vi "OEE_SCREEN_1_edit_running_summary.vi"(8 "error_in":errorcluster, 11 "running_summary":string) -> (0 "error_out":errorcluster, 3 "running_summary_updated":string)   [LabVIEW 2019]
uses:
  FGV/SQL_connection/FGV_OEE_SQL_connection.ctl
  FGV/SQL_raw_data/FGV_OEE_SQL_raw_data.ctl
  _misc/AULocalize/SubVIs/RegisterVI.vi
  _misc/AULocalize/SubVIs/Get Localized Phrase Compact Interface 0D.vi
panel:
  in  "summary_edit_cancel":bool caption="cancel"
  in  "summary_edit_update":bool caption="update"
  in  "running_summary_editor":string
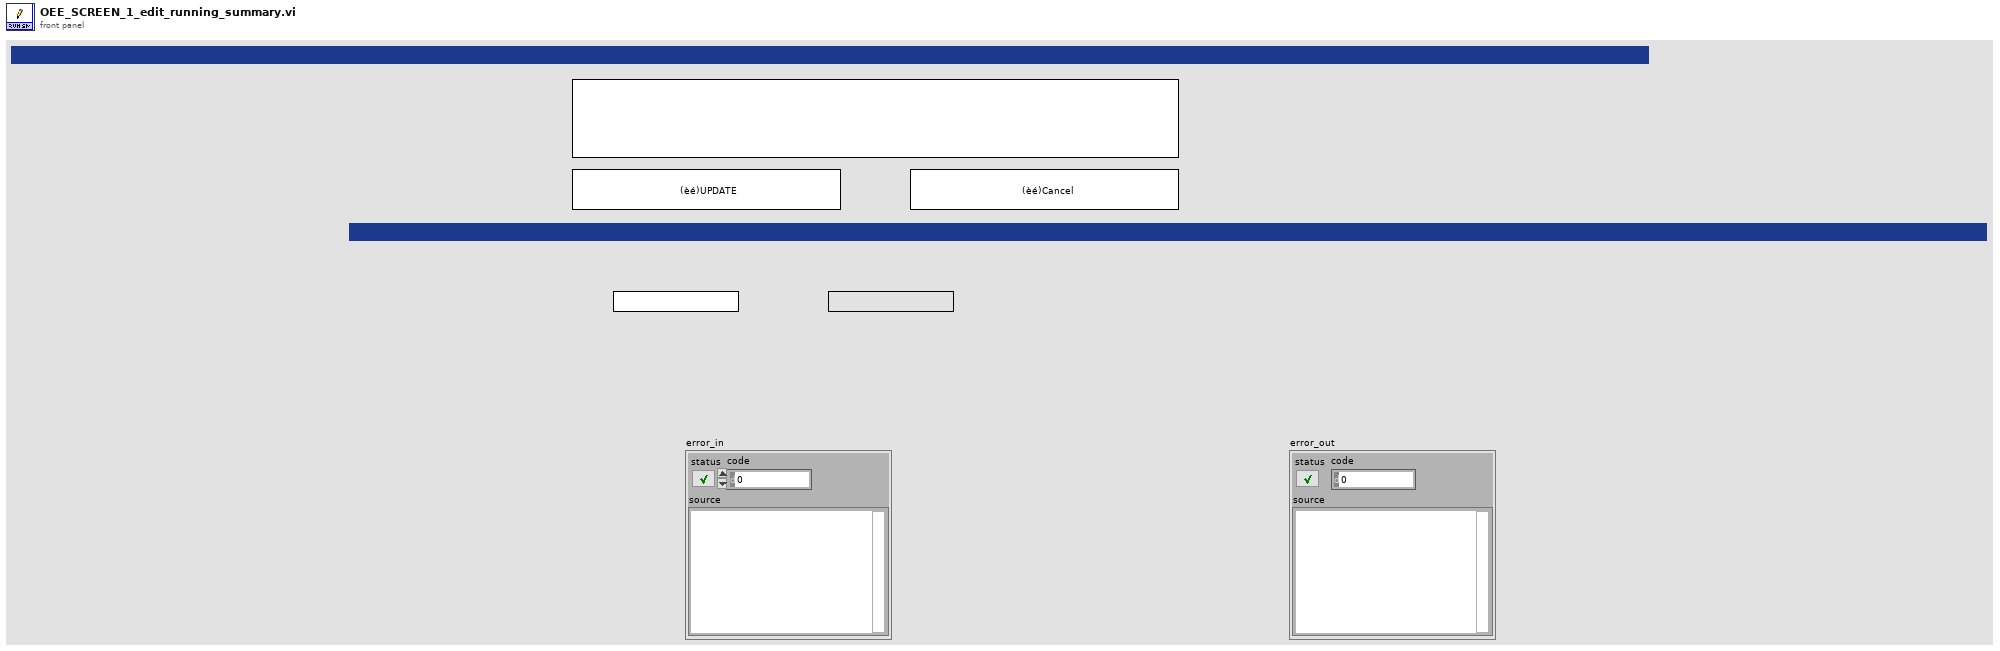
[diagram p1: front panel]
types:
  T1 = typedef "FGV_OEE_SQL_raw_data.ctl" = enum16{"initialize", "set_reference_name", "set_timestamp", "set_OK_NOK_count", "set_config_info", "set_pace", "set_availability", "set_hourly_ok_count", "set_targets", "get_all_info"}
  T2 = typedef "FGV_OEE_SQL_connection.ctl" = enum16{"initialize", "connect", "read_tables", "read_columns", "SELECT", "INSERT", "UPDATE", "DELETE", "EXEC + headers", "EXEC", "TRANSACTION", "connection_active?", "disconnect"}
  T3 = typedef "OEE_SQL_raw_data.ctl" = cluster{"reference_name":string, "data_timestamp":timestamp, "OK_NOK_count":string[][], "config_info":string[], "pace":string[][], "availability":string[], "hourly_ok_count":string[][], "shift_number":i8, "shift_start":i8, "shift_end":i8, "TAKT":u16, "FTTH_target":u16, "BOTTLENECK_station":string, "targets_hourly":u16[], "target_shift":u16}
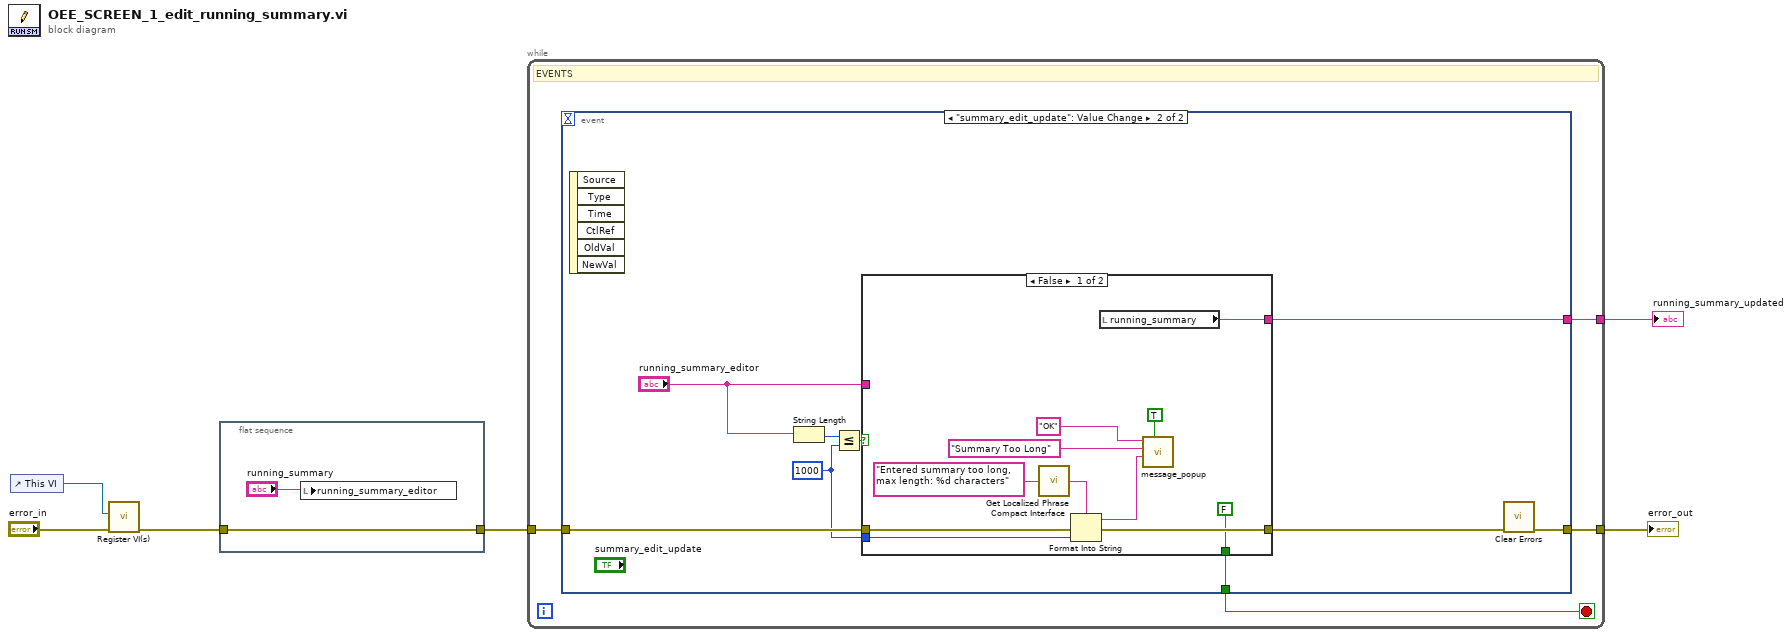
[diagram p0: block diagram]
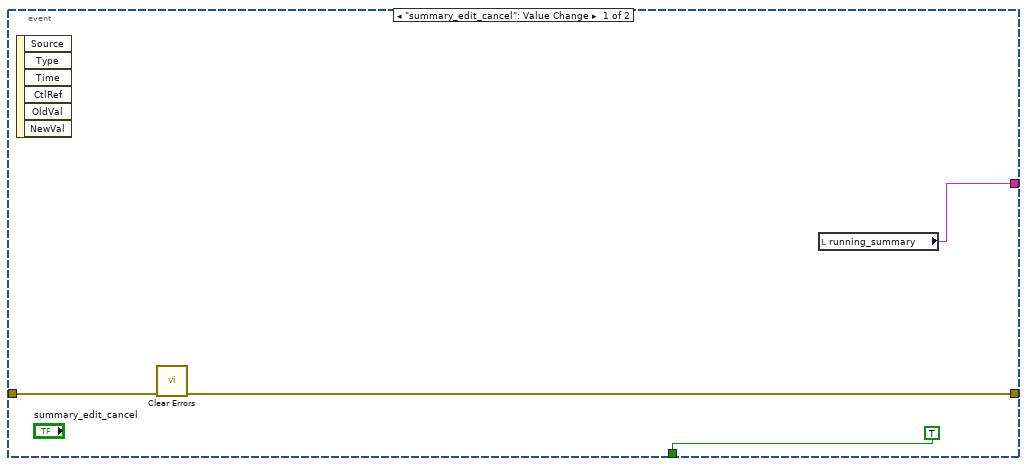
[diagram p2: hidden frame]
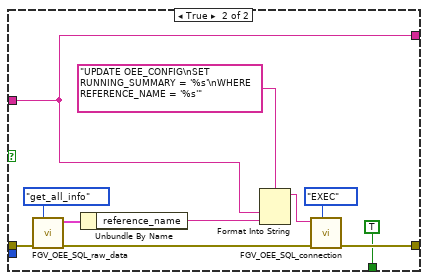
[diagram p3: hidden frame]
diagram:
  n1 = control-ref of="This VI"() -> (w1:refnum<vi>)
  n2 = call-poly "Register VI(s).vi"("error in"="error_in", "VI Ref"=w1) -> ("error out"=w2:errorcluster)  [unwired: 8 in, 1 out]
  n3 = flat-sequence {
    tunnel: w2 -> [w7]
    tunnel: [w7] -> w5
    frame #0 {
      n4 = local write "running_summary_editor"("running_summary") -> ()
    }
  }
  n5 = while {
    tunnel: w5 -> [w10]
    tunnel: [w12] -> w6
    tunnel: [w9] -> w4
    stop <- w11 stop-if-true
    # "EVENTS"
    n6 = event shown="[1] \"summary_edit_update\": Value Change" {
      selector: _ -> [_ _]
      dyn-events: _ -> [_ _]
      timeout: _ -> [_ _]
      tunnel: w10 -> [w15 w24]
      tunnel: [w14 w25] -> w12
      tunnel: [TRUE w18] -> w11
      tunnel: [w13 w17] -> w9
      event "summary_edit_cancel": Value Change {
        n7 = event-data() -> ()  [unwired: 1 in, 6 out]
        n8 = call <vilib>:"Clear Errors.vi"("error in (no error)"=w15) -> ("error out"=w14:errorcluster)  [unwired: 5 in, 1 out]
        n9 = local read "running_summary"() -> (w13:string)
      }
      event "summary_edit_update": Value Change {
        w20 = 1000 ("y")
        n10 = event-data() -> ()  [unwired: 1 in, 6 out]
        n11 = String Length(string="running_summary_editor") -> (length=w22:i32)
        n12 = Less Or Equal?(x=w22, y=w20) -> (x <= y?=w21:bool)
        n13 = case shown="False" w21 {
          tunnel: w24 -> [w33 w43]
          tunnel: [w32 w47] -> w23
          tunnel: w20 -> [w30 _]
          tunnel: "running_summary_editor" -> [_ w37]
          tunnel: [FALSE TRUE] -> w18
          tunnel: [w27 w37] -> w17
          frame False {
            n14 = call-poly "Get Localized Phrase Compact Interface.vi"("Key"="Entered summary too long, max length: %d characters" ("Message")) -> ("Translated Phrase"=w26:string)
            n15 = Format Into String(format string=w26, error in=w33, w30) -> (resulting string=w29:string, error out=w32:errorcluster)  [unwired: 1 in]
            n16 = local read "running_summary"() -> (w27:string)
            n17 = call "message_popup.vi"("Warning(T)/Info(F)"=TRUE, "Message"=w29, "Title"="Summary Too Long", "Button Label"="OK") -> ()  [unwired: 7 in, 1 out]
          }
          frame True {
            n18 = call "FGV_OEE_SQL_raw_data.vi"("options"=FGV_OEE_SQL_raw_data."get_all_info", "error_in"=w43) -> ("error_out"=w42:errorcluster, "SQL_raw_data_out"=w44:T3)  [unwired: 8 in]
            n19 = Unbundle By Name(w44) -> ("reference_name"=w40:string)
            n20 = Format Into String(format string="UPDATE OEE_CONFIG\nSET RUNNING_SUMMARY = '%s'\nWHERE REFERENCE_NAME = '%s'", w37, w40) -> (resulting string=w39:string)  [unwired: 2 in, 1 out]
            n21 = call "FGV_OEE_SQL_connection.vi"("options"=FGV_OEE_SQL_connection."EXEC", "error_in"=w42, "SQL_statement"=w39) -> ("error_out"=w47:errorcluster)  [unwired: 4 in, 4 out]
          }
        }
        n22 = call <vilib>:"Clear Errors.vi"("error in (no error)"=w23) -> ("error out"=w25:errorcluster)  [unwired: 5 in, 1 out]
      }
    }
  }
  "error_out" <- w6
  "running_summary_updated" <- w4
